vi "Populate Subpanels.vi"(8 "error in (no error)":errorcluster, 9 "View Labels (optional)":string[](array[string]), 10 "Views":refnum<class "Message Enqueuer.lvclass">[](array[class]), 11 "IModel In":refnum<class "IModel.lvclass">) -> (0 "error out":errorcluster, 3 "IModel Out":refnum<class "IModel.lvclass">)   [LabVIEW 2015, in "IModel.lvlib" / "IModel.lvclass"]
uses:
  IModel.lvclass
  <vilib>/ActorFramework/Message Enqueuer/Message Enqueuer.lvclass
  IModel.lvclass/IModel.ctl
  IViewable/IViewable Messages/Insert View Msg/Insert View Msg.lvclass/Insert View Msg.ctl
  <vilib>/ActorFramework/Message Enqueuer/Message Enqueuer.lvclass/Message Enqueuer.ctl
  <vilib>/ActorFramework/Message Enqueuer/Enqueue.vi
  <vilib>/ActorFramework/Message Priority Queue/Priority Enqueue.vi
  IViewManager/IViewManager/IViewManager.lvclass
  IViewable/IViewable Messages/Insert View Msg/Insert View Msg.lvclass
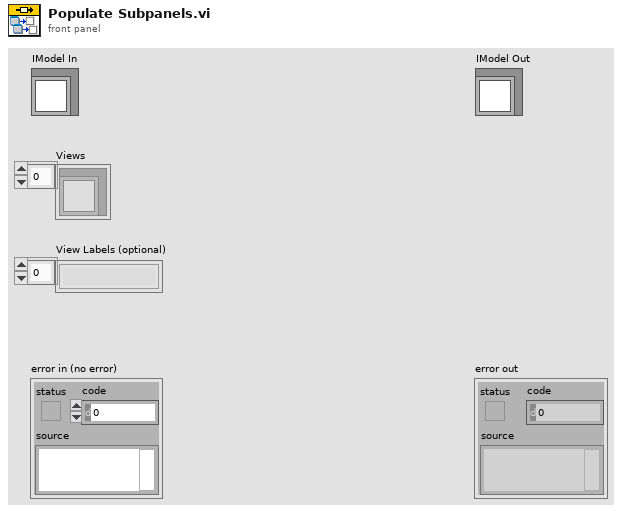
[diagram p1: front panel]
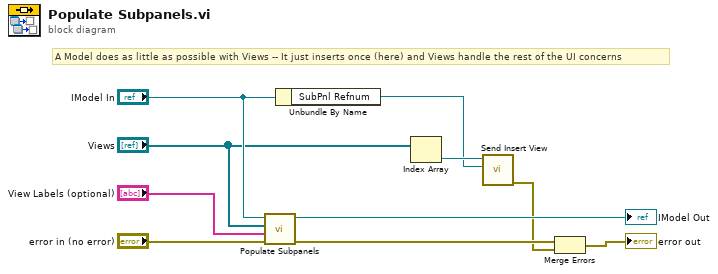
[diagram p0: block diagram]
diagram:
  # "A Model does as little as possible with Views -- It just inserts once (here) and Views handle the rest of the UI concerns"
  n1 = call-parent "Populate Subpanels.vi"("error in (no error)"="error in (no error)", "View Labels (optional)"="View Labels (optional)", "Views"="Views", "IViewManager In"="IModel In") -> ("error out"=w10:errorcluster, "IViewManager Out"=→"IModel Out":refnum<class "IModel.lvclass">)  [unwired: 6 in]
  n2 = Unbundle By Name("IModel In") -> ("SubPnl Refnum"=w3:refnum<vi>)
  n3 = Index Array(array="Views") -> (element=w4:refnum<class "Message Enqueuer.lvclass">)  [unwired: 1 in]
  n4 = call "Send Insert View.vi"("SubPnl Refnum"=w3, "Message Enqueuer"=w4) -> ("error out"=w1:errorcluster)  [unwired: 8 in, 1 out]
  n5 = Merge Errors(w10, w1) -> (→"error out":errorcluster)
